vi "GetSettings_WithDefinedName_ReturnsConfiguredValue.vi"(9 "Expected":string="Test.lvlib", 10 "Name":string="ProjectLibrarySuffix", 11 "Content":string="[LVUnit]\nProjectLibrarySuffix=Test.lvlib\nDeferDrawingDuringTest=True") -> (0 "error out":errorcluster)   [LabVIEW 2017, in "ConfigurationTest.lvlib"]
uses:
  ConfigurationTest.lvlib
  98bcd5d9-f4f5-4994-9e08-55a29551327a.vi
  Constraint/IsEqual/Create.vi
  Constraint/IsEqual/IsEqual.lvclass
  Configuration/Configuration.lvlib
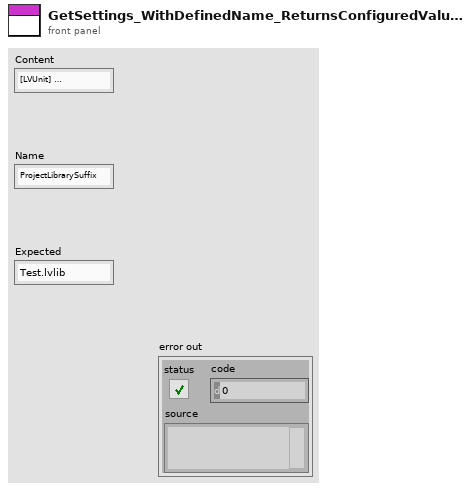
[diagram p1: front panel]
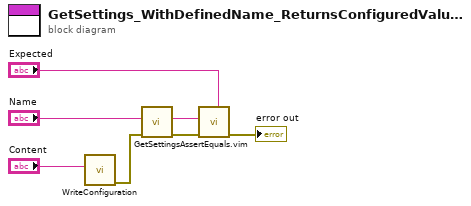
[diagram p0: block diagram]
diagram:
  n1 = call "WriteConfiguration.vi"("Content"="Content") -> ("error out"=w2:errorcluster)  [unwired: 10 in]
  n2 = call "GetSettings.vi"("error in (no error)"=w2, "Name"="Name") -> ("error out"=w6:errorcluster, "Value"=w5:string)  [unwired: 8 in]
  n3 = call "AssertEquals.vim"("Expected"="Expected", "error in (no error)"=w6, "Actual"=w5) -> ("error out"=→"error out":errorcluster)  [unwired: 8 in]
